vi "Resize Pane.vi"(6 "Pane size":i32, 8 "error in (no error)":errorcluster, 11 "IContainer in":refnum<class "IContainer.lvclass">) -> (0 "error out":errorcluster, 2 "Resized?":bool, 3 "IContainer out":refnum<class "IContainer.lvclass">)   [LabVIEW 2021, in "IContainer.lvclass"]
doc: "Copyright 2018, Wiebe Walstra, wiebe@carya.nl."
uses:
  IContainer.lvclass
  IContainer.lvclass/IContainer.ctl
  IObject.lvclass
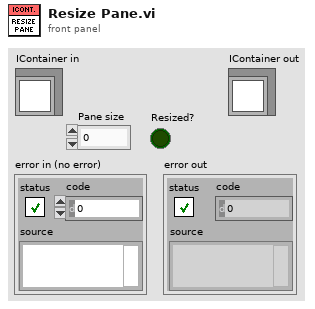
[diagram p1: front panel]
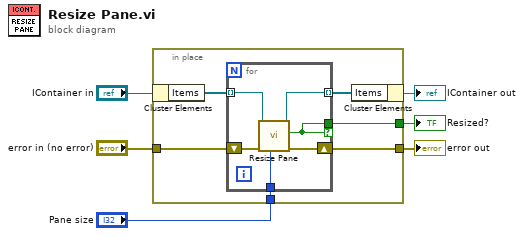
[diagram p0: block diagram]
diagram:
  n1 = in-place {
    in-place-border: [w12] -> w6
    in-place-border: "Pane size" -> [w11]
    in-place-border: "error in (no error)" -> [w10]
    in-place-border: [w7] -> w1
    n2 = in-place-cluster #1("IContainer in") -> ("Items"=w9:refnum<class "IObject.lvclass">[])
    n3 = for {
      tunnel: [w17] -> w8 mode=indexing
      tunnel: w11 -> [w16]
      tunnel: w9 -> [w14] mode=indexing
      shift-right: [w18] -> w12
      shift-left: w10 -> [w15]
      tunnel: [w13] -> w7 if=w13
      n4 = call-dynamic "Resize Pane.vi"("Pane size"=w16, "error in (no error)"=w15, "IObject in"=w14) -> ("error out"=w18:errorcluster, "Resized?"=w13:bool, "IObject out"=w17:refnum<class "IObject.lvclass">)  [unwired: 6 in]
    }
    n5 = in-place-cluster #1("Items"=w8) -> (→"IContainer out":refnum<class "IContainer.lvclass">)
  }
  "error out" <- w6
  "Resized?" <- w1
